vi "DIMAQ LoopThroughImageFolder.vi"() -> ()   [LabVIEW 2014]
panel:
  out "?":T1(plugin-control)
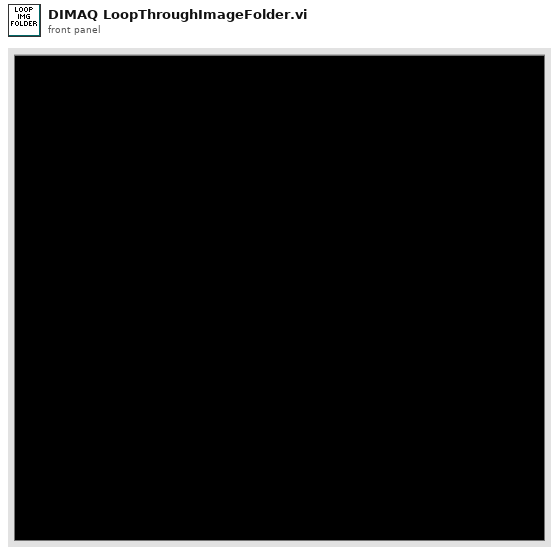
[diagram p1: front panel]
types:
  T1 = typedef "IMAQ Image.ctl" = refnum<image>
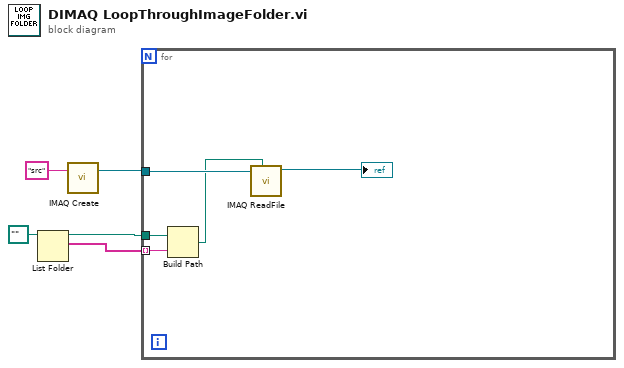
[diagram p0: block diagram]
diagram:
  n1 = List Folder(path=path "") -> (path out=w2:path, filenames=w1:string[])  [unwired: 3 in, 2 out]
  n2 = call "IMAQ Create"("Image Name"="src") -> ("New Image"=w3:T1)  [unwired: 4 in, 1 out]
  n3 = for {
    tunnel: w3 -> [w10]
    tunnel: w2 -> [w9]
    tunnel: w1 -> [w8] mode=indexing
    n4 = Build Path(base path=w9, name or relative path=w8) -> (appended path=w7:path)
    n5 = call "IMAQ ReadFile"("File Path"=w7, "Image"=w10) -> ("Image Out"=→"?":T1)  [unwired: 5 in, 4 out]
  }
